vi "Project Parser_Class Array.vi"(6 "To Lower Case?(T)":bool=TRUE, 7 "Load Stored Targets?(T)":bool=TRUE, 8 "Error In":errorcluster, 10 "Dependency Source Plugins":refnum<class "Dependency Source.lvclass">[](array[class]), 11 "Project Path in":path) -> (0 "Error Out":errorcluster, 1 "Found External Dependencies":T1[](array[typedef]), 2 "Found Internal Dependencies":T1[](array[typedef]), 3 "Project Path dub":path, 4 "Unhandled Targets":T1[](array[typedef]), 5 "Plugin Load Success? Array":bool[](array[boolean]))   [LabVIEW 2019, in "Project.Dependencies Finder.lvlib"]
doc: "Parse a project file for internal and external dependencies.\n\nInternal dependencies are expected to have 'paths' like vi.lib\\ and should be found inside the LabVIEW folder.\nExternal dependencies are identified by unique folder names.\n\n2020-11-13: Henrik Dueholm Hansen"
uses:
  Project.Dependencies Finder.lvlib
  Ctl/Ctl_Dependency Element.ctl
  Dependency Source/Dependency Source.lvclass
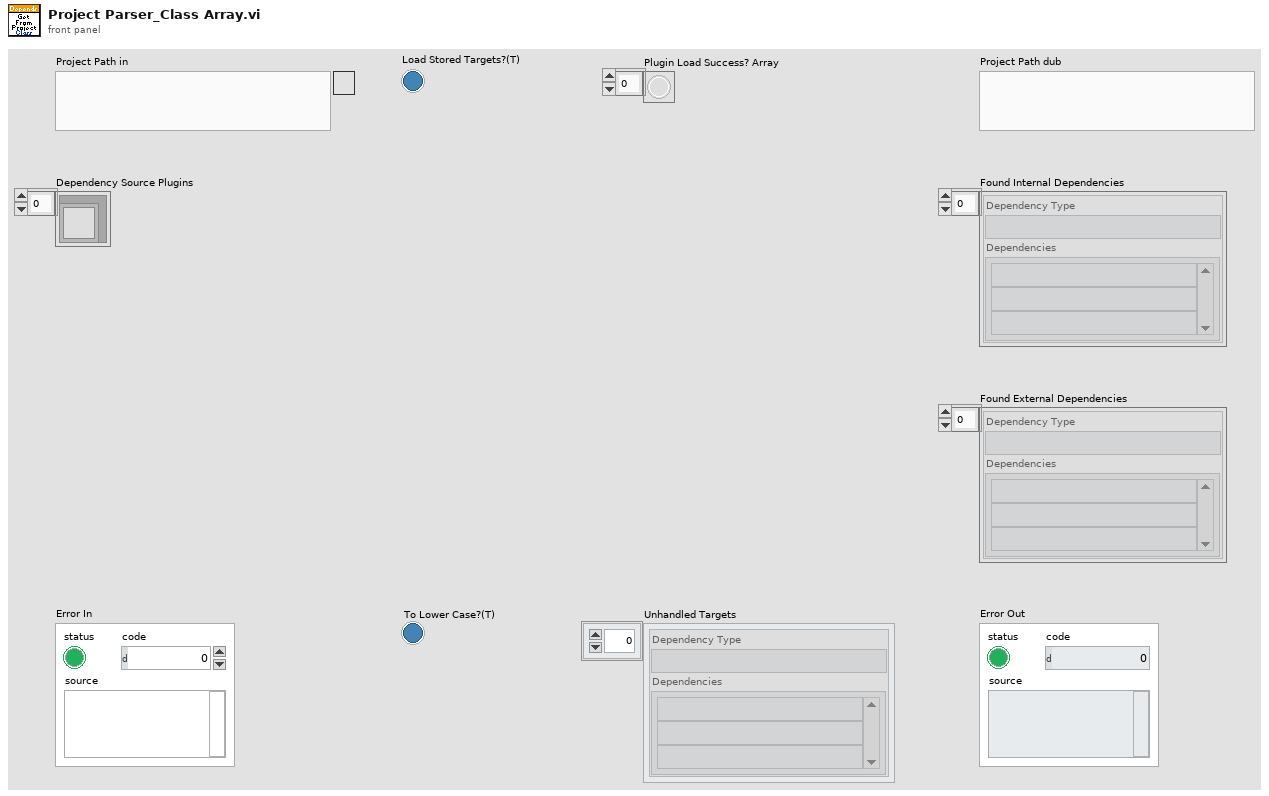
[diagram p1: front panel]
types:
  T1 = typedef "Project.Dependencies Finder.lvlib/Ctl_Dependency Element.ctl" = cluster{"Dependency Type":string, "Dependencies":string[]}
  T2 = typedef "Project.Dependencies Finder.lvlib/Ctl_External Target Element.ctl" = cluster{"Target Source":string, "External Target Map":map{string, string}}
  T3 = typedef "Project.Dependencies Finder.lvlib/Ctl_Internal Target Element.ctl" = cluster{"Target Source":string, "Internal Target Map":map{string, string}}
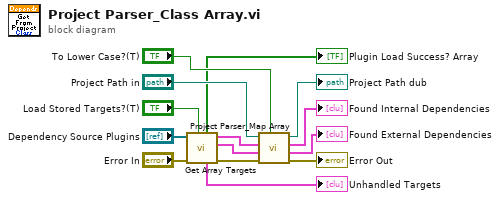
[diagram p0: block diagram]
diagram:
  n1 = call "Get Array Targets.vi"("Load Stored Targets?(T)"="Load Stored Targets?(T)", "error in (no error)"="Error In", "Dependency Sources"="Dependency Source Plugins") -> ("error out"=w9:errorcluster, "External Targets"=w10:T2[], "Internal Targets"=w11:T3[], "Unhandled Targets"=→"Unhandled Targets":T1[], "Success? Array"=→"Plugin Load Success? Array":bool[])  [unwired: 3 in, 1 out]
  n2 = call "Project Parser_Map Array.vi"("To Lower Case?(T)"="To Lower Case?(T)", "Error In"=w9, "External Targets"=w10, "Internal Targets"=w11, "Project Path in"="Project Path in") -> ("Error Out"=→"Error Out":errorcluster, "Found External Dependencies"=→"Found External Dependencies":T1[], "Found Internal Dependencies"=→"Found Internal Dependencies":T1[], "Project Path dub"=→"Project Path dub":path)  [unwired: 3 in]
